vi "Launch Topic.vi"(7 "Include Initial Value? (F)":bool, 9 "Type":variant, 10 "Datum Name":string, 11 "Mediator in":refnum<class "Mediator.lvclass">) -> (0 "error out":errorcluster, 2 "New Topic Enqueuer":refnum<class "Message Enqueuer.lvclass">, 3 "Mediator out":refnum<class "Mediator.lvclass">)   [LabVIEW 2015, in "Mediator.lvlib" / "Mediator.lvclass"]
uses:
  Mediator.lvclass
  <vilib>/ActorFramework/Message Enqueuer/Message Enqueuer.lvclass
  Mediator.lvclass/Mediator.ctl
  SubscriptionPolicy/ValueChangeSubscription/ValueChangeSubscription.lvclass/ValueChangeSubscription.ctl
  Topic Messages/Add Topic Subscriber Msg/Add Topic Subscriber Msg.lvclass/Add Topic Subscriber Msg.ctl
  <vilib>/ActorFramework/Message Enqueuer/Message Enqueuer.lvclass/Message Enqueuer.ctl
  <vilib>/ActorFramework/Message Enqueuer/Enqueue.vi
  <vilib>/ActorFramework/Message Priority Queue/Priority Enqueue.vi
  SubscriptionPolicy/ValueChangeSubscription/ValueChangeSubscription.lvclass
  Topic Messages/Add Topic Subscriber Msg/Add Topic Subscriber Msg.lvclass
  Topic/Topic.lvclass
  <vilib>/ActorFramework/Actor/Actor.lvclass
  TopicLookupTable/TopicLookupTable.lvclass
  IMediator/ISubscriptionPolicy/ISubscriptionPolicy.lvclass
  IObserver/ActorDataBinding/ActorDataBinding.lvclass
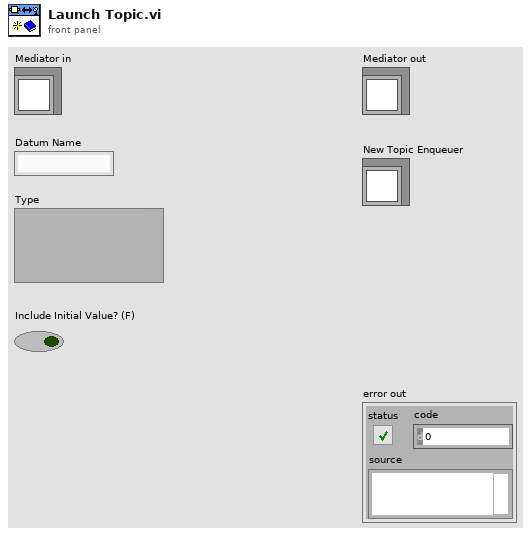
[diagram p1: front panel]
types:
  T1 = typedef "IMediator.lvlib/ISubscriptionPolicy.lvclass/ISubscriptionPolicy Reference.ctl" = refnum<data-value>
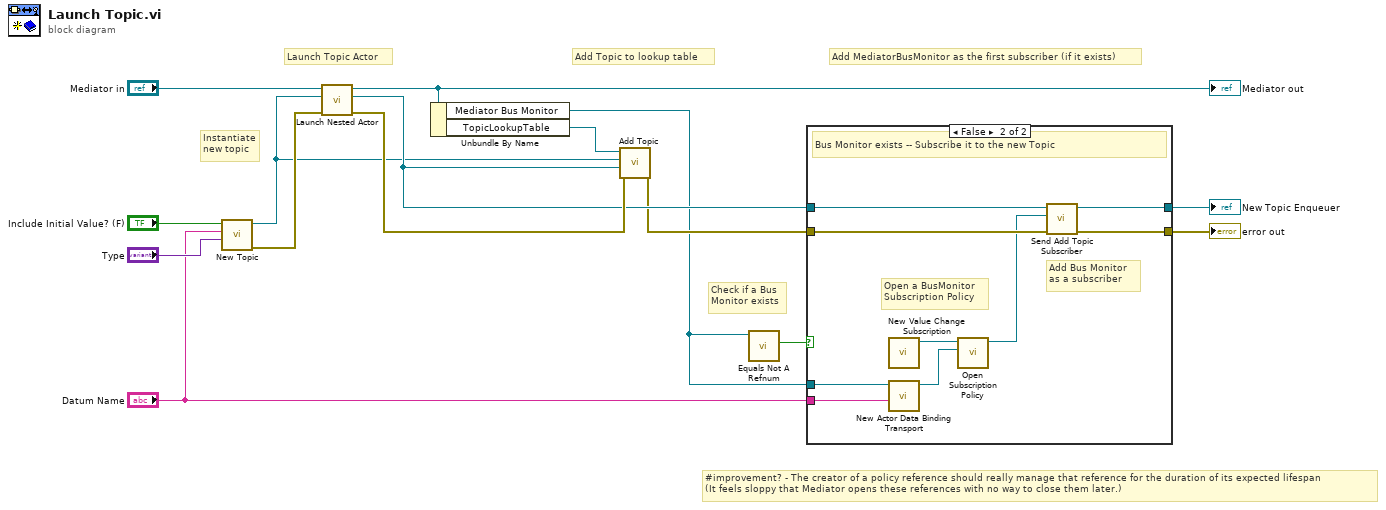
[diagram p0: block diagram]
diagram:
  # "Check if a Bus\nMonitor exists"
  # "#improvement? - The creator of a policy reference should really manage that reference for the duration of its expected lifespan\n(It feels sloppy that Mediator opens these references with no way to close them later.)"
  # "Add MediatorBusMonitor as the first subscriber (if it exists)"
  # "Launch Topic Actor"
  # "Add Topic to lookup table"
  # "Instantiate\nnew topic"
  n1 = call "New Topic.vi"("New Topic Data"="Type", "Name"="Datum Name", "Use Type Input As Initial Value?"="Include Initial Value? (F)") -> ("error out"=w9:errorcluster, "Topic out"=w8:refnum<class "Topic.lvclass">)  [unwired: 7 in]
  n2 = call <vilib>:"Launch Nested Actor.vi"("error in (no error)"=w9, "Nested Actor"=w8, "Caller Actor in"="Mediator in") -> ("error out"=w12:errorcluster, "Nested Actor's Enqueuer"=w10:refnum<class "Message Enqueuer.lvclass">, "Caller Actor out"=w4:refnum<class "Mediator.lvclass">)  [unwired: 6 in]
  "Mediator out" <- w4
  n3 = Unbundle By Name(w4) -> ("Mediator Bus Monitor"=w1:refnum<class "Message Enqueuer.lvclass">, "TopicLookupTable"=w7:refnum<data-value>)
  n4 = call "Add Topic.vi"("error in (no error)"=w12, "Topic Enqueuer"=w10, "Topic Object"=w8, "TopicLookupTable"=w7) -> ("error out"=w6:errorcluster)  [unwired: 5 in, 2 out]
  n5 = call <vilib>:"Equals Not A Refnum.vi"("Message Enqueuer"=w1) -> ("Not a refnum?"=w3:bool)  [unwired: 10 in]
  n6 = case shown="False" w3 {
    tunnel: "Datum Name" -> [_ w19]
    tunnel: [w17 w24] -> w11
    tunnel: w10 -> [w17 w23]
    tunnel: w6 -> [w16 w22]
    tunnel: [w16 w21] -> w5
    tunnel: w1 -> [_ w20]
    frame True {
      # "Actor queue = Not a refnum -- Bus Monitor does not exist"
    }
    frame False {
      # "Open a BusMonitor\nSubscription Policy"
      # "Add Bus Monitor\nas a subscriber"
      # "Bus Monitor exists -- Subscribe it to the new Topic"
      n7 = call "New Value Change Subscription.vi"() -> ("ValueChangeSubscription Out"=w25:refnum<class "ValueChangeSubscription.lvclass">)  [unwired: 11 in]
      n8 = call "New Actor Data Binding Transport.vi"("Datum Return Name"=w19, "IObserver"=w20) -> ("ActorDataBinding out"=w26:refnum<class "ActorDataBinding.lvclass">)  [unwired: 8 in, 1 out]
      n9 = call "Open Subscription Policy.vi"("Transport"=w26, "SubscriptionPolicy"=w25) -> ("Subscription Policy"=w18:T1)  [unwired: 8 in, 1 out]
      n10 = call "Send Add Topic Subscriber.vi"("error in (no error)"=w22, "Subscription Policy"=w18, "Message Enqueuer"=w23) -> ("error out"=w21:errorcluster, "Message Enqueuer out"=w24:refnum<class "Message Enqueuer.lvclass">)  [unwired: 7 in]
    }
  }
  "error out" <- w5
  "New Topic Enqueuer" <- w11
